vi "Nigel Tamagotchi Main.vi"() -> ()   [LabVIEW 2026]
uses:
  Type Defs/Queue Data.ctl
  Type Defs/Handler Data.ctl
panel:
  in  "Stop":bool
  out "Age (cycles)":u32
  out "Mood":string
  out "Cleanliness":i16(slide)=100 scale=0.0..100.0
  out "Energy":i16(slide)=100 scale=0.0..100.0
  out "Hunger":i16(slide) scale=0.0..100.0
  in  "Fixed Bug Button":bool
  in  "Broken Arrow Button":bool
  in  "Spagetti Button":bool
  in  "Sleep Button":bool
  in  "Clean Button":bool
  in  "Feed Button":bool
  out "Pict Ring":u16(ring)
  # "Nigel-gotchi (QMH)"
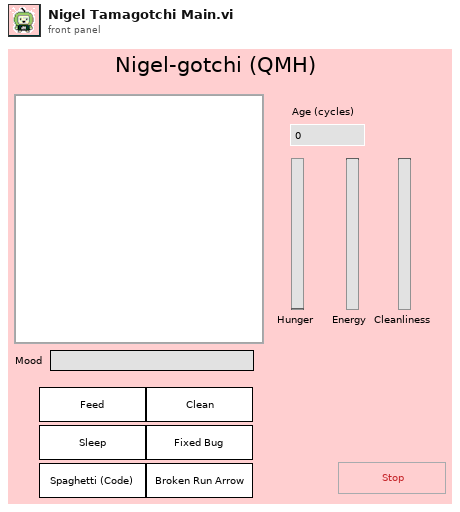
[diagram p1: front panel]
types:
  T1 = typedef "Queue Data.ctl" = cluster{"State":string, "Data":variant}
  T2 = typedef "Handler Data.ctl" = cluster{"Age (cycles)":u32, "Mood Override Counter":u32, "Mood Override":string, "Energy":i16, "Hunger":i16, "Cleanliness":i16}
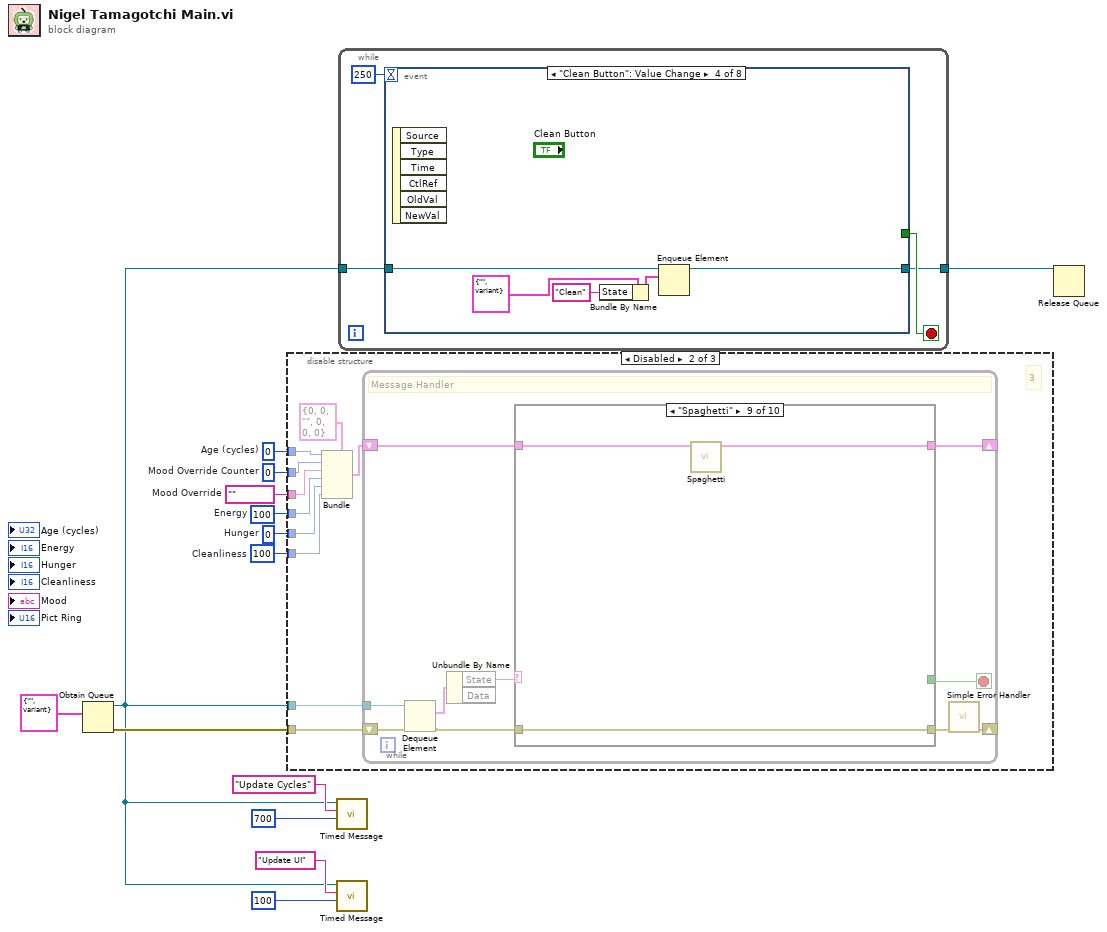
[diagram p0: block diagram]
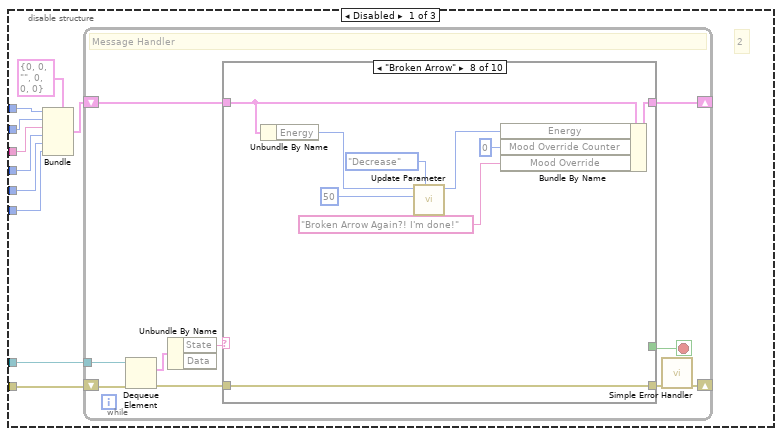
[diagram p2: hidden frame]
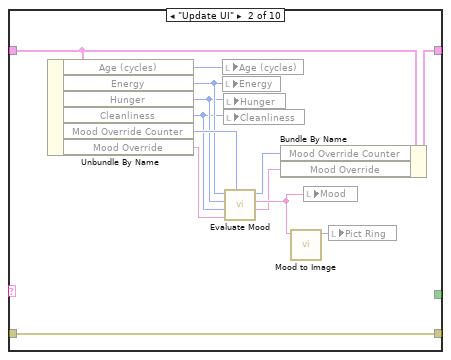
[diagram p4: hidden frame]
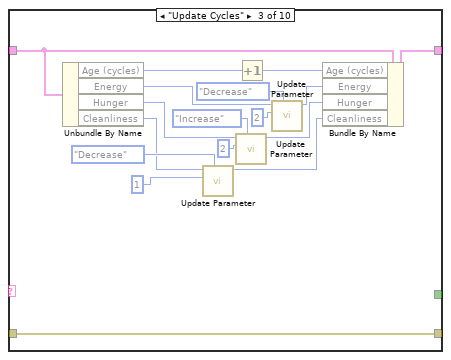
[diagram p5: hidden frame]
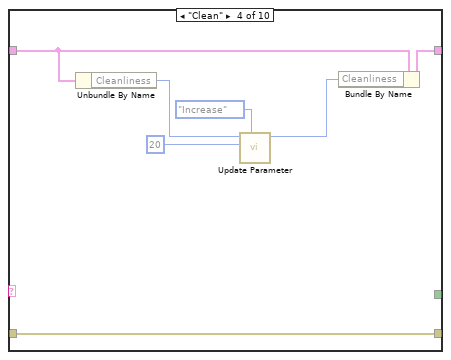
[diagram p6: hidden frame]
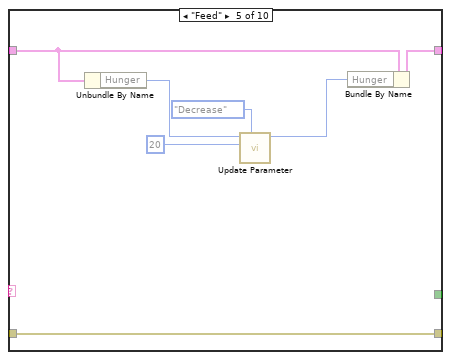
[diagram p7: hidden frame]
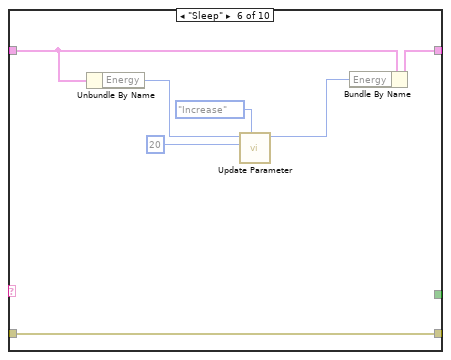
[diagram p8: hidden frame]
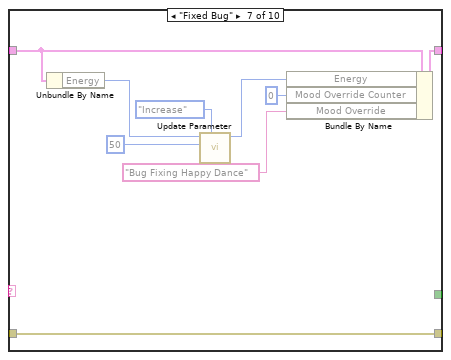
[diagram p9: hidden frame]
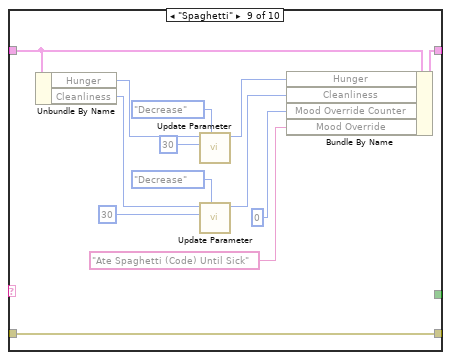
[diagram p10: hidden frame]
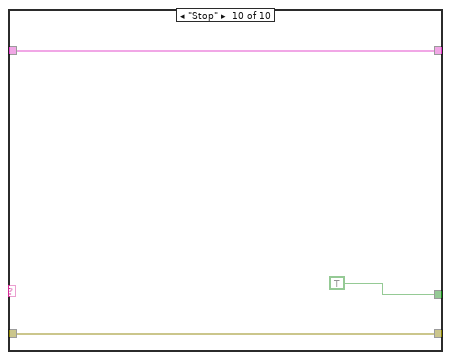
[diagram p11: hidden frame]
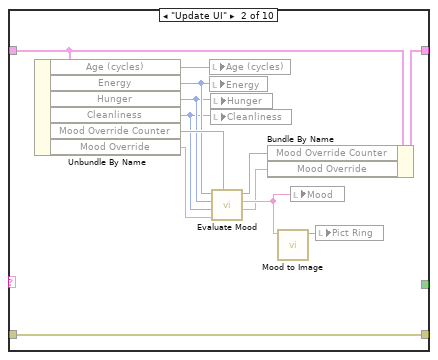
[diagram p13: hidden frame]
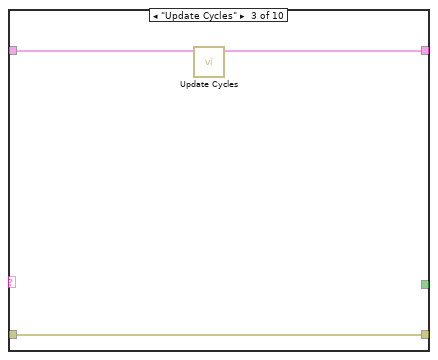
[diagram p14: hidden frame]
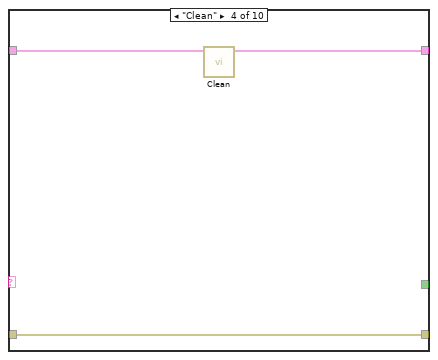
[diagram p15: hidden frame]
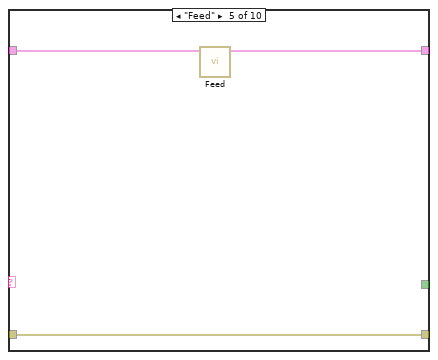
[diagram p16: hidden frame]
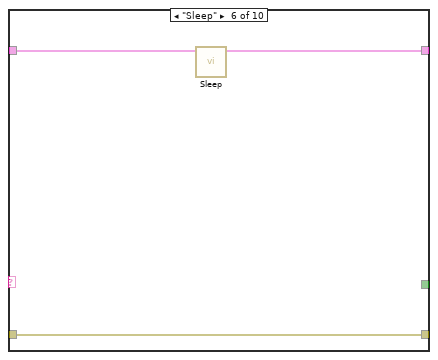
[diagram p17: hidden frame]
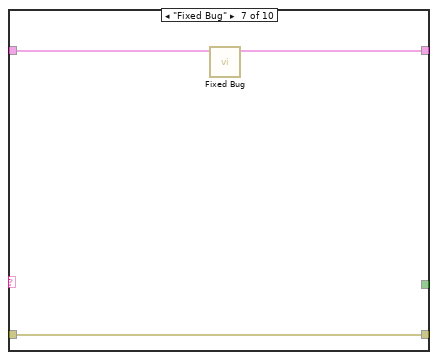
[diagram p18: hidden frame]
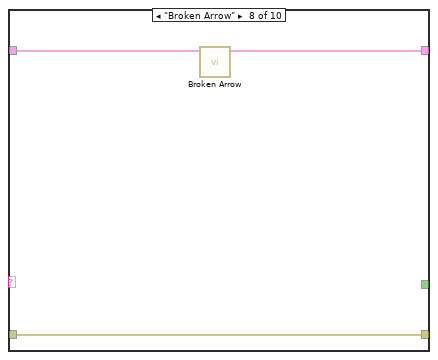
[diagram p19: hidden frame]
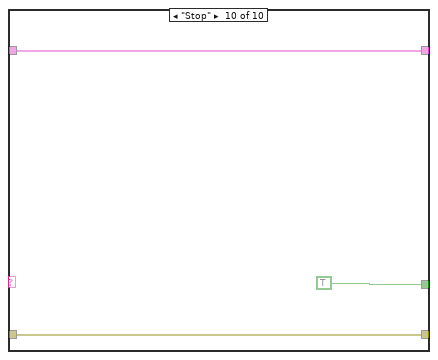
[diagram p20: hidden frame]
diagram:
  w7 = u32 0  # Mood Override Counter
  w10 = i16 100  # Energy
  w8 = i16 100  # Cleanliness
  w12 = u32 0  # Age (cycles)
  w9 = i16 0  # Hunger
  w11 = ""  # Mood Override
  n1 = Obtain Queue(element data type=T1 {"State"="", "Data"=variant}) -> (queue out=w1:refnum<queue>, error out=w13:errorcluster)  [unwired: 4 in, 1 out]
  n2 = disable-structure shown="Disabled" {
    disable-tunnel: w13 -> [w24 w131 w188]
    disable-tunnel: w12 -> [w22 w129 w187]
    disable-tunnel: w11 -> [w20 w127 w186]
    disable-tunnel: w10 -> [w19 w126 w185]
    disable-tunnel: w9 -> [w18 w125 w184]
    disable-tunnel: w8 -> [w17 w124 w183]
    disable-tunnel: w7 -> [w21 w128 w182]
    disable-tunnel: w1 -> [w23 w130 w181]
    frame Disabled {
      # "2"
      n3 = Bundle(cluster=T2 {"Age (cycles)"=0, "Mood Override Counter"=0, "Mood Override"="", "Energy"=0, "Hunger"=0, "Cleanliness"=0}, "Age (cycles)"=w22, "Mood Override Counter"=w21, "Mood Override"=w20, "Energy"=w19, "Hunger"=w18, "Cleanliness"=w17) -> (w16:T2)
      n4 = while {
        tunnel: w23 -> [w34]
        shift-right: [w29] -> _
        shift-left: w16 -> [w28]
        shift-right: [w25] -> _
        shift-left: w24 -> [w33]
        stop <- w30 stop-if-true
        # "Message Handler"
        n5 = Dequeue Element(queue=w34, error in (no error)=w33) -> (element=w32:T1, error out=w27:errorcluster)  [unwired: 1 in, 2 out]
        n6 = Unbundle By Name(w32) -> ("State"=w31:string)  [unwired: 1 out]
        n7 = case shown="\"Broken Arrow\"" w31 {
          tunnel: [_ _ _ _ _ _ _ _ _ TRUE] -> w30
          tunnel: [w36 w45 w58 w68 w75 w82 w91 w100 w113 w120] -> w29
          tunnel: w28 -> [w36 w47 w60 w70 w77 w84 w93 w102 w115 w120]
          tunnel: w27 -> [w35 w37 w50 w67 w74 w81 w88 w97 w106 w119]
          tunnel: [w35 w37 w50 w67 w74 w81 w88 w97 w106 w119] -> w26
          frame Default {
          }
          frame "Update UI" {
            # "Update UI (and cycles every tenth refresh)"
            n8 = Unbundle By Name(w47) -> ("Age (cycles)"=w46:u32, "Energy"=w40:i16, "Hunger"=w39:i16, "Cleanliness"=w38:i16, "Mood Override Counter"=w42:u32, "Mood Override"=w41:string)
            n9 = local write "Age (cycles)"(w46) -> ()
            n10 = local write "Energy"(w40) -> ()
            n11 = local write "Hunger"(w39) -> ()
            n12 = local write "Cleanliness"(w38) -> ()
            n13 = call "Evaluate Mood.vi"("Mood Override Counter"=w42, "Override Mood"=w41, "Cleanliness"=w38, "Hunger"=w39, "Energy"=w40) -> ("Mood Override"=w44:string, "Mood"=w49:string, "Mood Override Counter out"=w43:u32)  [unwired: 4 in]
            n14 = Bundle By Name(cluster=w47, "Mood Override Counter"=w43, "Mood Override"=w44) -> (w45:T2)
            n15 = call "Mood to Image.vi"("Mood"=w49) -> ("Image number"=w48:u16)  [unwired: 10 in]
            n16 = local write "Mood"(w49) -> ()
            n17 = local write "Pict Ring"(w48) -> ()
          }
          frame "Update Cycles" {
            n18 = Unbundle By Name(w60) -> ("Age (cycles)"=w59:u32, "Energy"=w56:i16, "Hunger"=w54:i16, "Cleanliness"=w52:i16)
            n19 = call "Update Parameter.vi"("Action"=enum16{"Increase", "Decrease"}."Decrease", "Modifier"=i16 1, "Parameter"=w52) -> ("New Value"=w51:i16)  [unwired: 8 in]
            n20 = call "Update Parameter.vi"("Action"=enum16{"Increase", "Decrease"}."Increase", "Modifier"=i16 2, "Parameter"=w54) -> ("New Value"=w53:i16)  [unwired: 8 in]
            n21 = Increment(x=w59) -> (x+1=w57:u32)
            n22 = call "Update Parameter.vi"("Action"=enum16{"Increase", "Decrease"}."Decrease", "Modifier"=i16 2, "Parameter"=w56) -> ("New Value"=w55:i16)  [unwired: 8 in]
            n23 = Bundle By Name(cluster=w60, "Age (cycles)"=w57, "Energy"=w55, "Hunger"=w53, "Cleanliness"=w51) -> (w58:T2)
          }
          frame "Clean" {
            # "Add 20, but make sure it doesn't go above 100 percent or below 0"
            n24 = Unbundle By Name(w70) -> ("Cleanliness"=w71:i16)
            n25 = call "Update Parameter.vi"("Action"=enum16{"Increase", "Decrease"}."Increase", "Modifier"=i16 20 ("y"), "Parameter"=w71) -> ("New Value"=w69:i16)  [unwired: 8 in]
            n26 = Bundle By Name(cluster=w70, "Cleanliness"=w69) -> (w68:T2)
          }
          frame "Feed" {
            # "Add 20, but make sure it doesn't go above 100 percent or below 0"
            n27 = Unbundle By Name(w77) -> ("Hunger"=w78:i16)
            n28 = call "Update Parameter.vi"("Action"=enum16{"Increase", "Decrease"}."Decrease", "Modifier"=i16 20 ("y"), "Parameter"=w78) -> ("New Value"=w76:i16)  [unwired: 8 in]
            n29 = Bundle By Name(cluster=w77, "Hunger"=w76) -> (w75:T2)
          }
          frame "Sleep" {
            # "Add 20, but make sure it doesn't go above 100 percent or below 0"
            n30 = Unbundle By Name(w84) -> ("Energy"=w85:i16)
            n31 = call "Update Parameter.vi"("Action"=enum16{"Increase", "Decrease"}."Increase", "Modifier"=i16 20 ("y"), "Parameter"=w85) -> ("New Value"=w83:i16)  [unwired: 8 in]
            n32 = Bundle By Name(cluster=w84, "Energy"=w83) -> (w82:T2)
          }
          frame "Fixed Bug" {
            n33 = Unbundle By Name(w93) -> ("Energy"=w94:i16)
            n34 = call "Update Parameter.vi"("Action"=enum16{"Increase", "Decrease"}."Increase", "Modifier"=i16 50 ("y"), "Parameter"=w94) -> ("New Value"=w92:i16)  [unwired: 8 in]
            n35 = Bundle By Name(cluster=w93, "Energy"=w92, "Mood Override Counter"=u32 0, "Mood Override"="Bug Fixing Happy Dance") -> (w91:T2)
          }
          frame "Broken Arrow" {
            n36 = Unbundle By Name(w102) -> ("Energy"=w103:i16)
            n37 = call "Update Parameter.vi"("Action"=enum16{"Increase", "Decrease"}."Decrease", "Modifier"=i16 50 ("y"), "Parameter"=w103) -> ("New Value"=w101:i16)  [unwired: 8 in]
            n38 = Bundle By Name(cluster=w102, "Energy"=w101, "Mood Override Counter"=u32 0, "Mood Override"="Broken Arrow Again?! I'm done!") -> (w100:T2)
          }
          frame "Spaghetti" {
            n39 = Unbundle By Name(w115) -> ("Hunger"=w116:i16, "Cleanliness"=w108:i16)
            n40 = call "Update Parameter.vi"("Action"=enum16{"Increase", "Decrease"}."Decrease", "Modifier"=i16 30 ("y"), "Parameter"=w116) -> ("New Value"=w114:i16)  [unwired: 8 in]
            n41 = call "Update Parameter.vi"("Action"=enum16{"Increase", "Decrease"}."Decrease", "Modifier"=i16 30 ("y"), "Parameter"=w108) -> ("New Value"=w107:i16)  [unwired: 8 in]
            n42 = Bundle By Name(cluster=w115, "Hunger"=w114, "Cleanliness"=w107, "Mood Override Counter"=u32 0, "Mood Override"="Ate Spaghetti (Code) Until Sick") -> (w113:T2)
          }
          frame "Stop" {
          }
        }
        n43 = call <vilib>:"Simple Error Handler.vi"("error in (no error)"=w26) -> ("error out"=w25:errorcluster)  [unwired: 4 in, 4 out]
      }
    }
    frame Disabled {
      # "3"
      n44 = Bundle(cluster=T2 {"Age (cycles)"=0, "Mood Override Counter"=0, "Mood Override"="", "Energy"=0, "Hunger"=0, "Cleanliness"=0}, "Age (cycles)"=w129, "Mood Override Counter"=w128, "Mood Override"=w127, "Energy"=w126, "Hunger"=w125, "Cleanliness"=w124) -> (w123:T2)
      n45 = while {
        tunnel: w130 -> [w141]
        shift-right: [w136] -> _
        shift-left: w123 -> [w135]
        shift-right: [w132] -> _
        shift-left: w131 -> [w140]
        stop <- w137 stop-if-true
        # "Message Handler"
        n46 = Dequeue Element(queue=w141, error in (no error)=w140) -> (element=w139:T1, error out=w133:errorcluster)  [unwired: 1 in, 2 out]
        n47 = Unbundle By Name(w139) -> ("State"=w138:string)  [unwired: 1 out]
        n48 = case shown="\"Spaghetti\"" w138 {
          tunnel: [_ _ _ _ _ _ _ _ _ TRUE] -> w137
          tunnel: [w143 w152 w158 w161 w164 w167 w170 w173 w175 w179] -> w136
          tunnel: w135 -> [w143 w154 w159 w162 w165 w168 w171 w174 w176 w179]
          tunnel: [w142 w144 w157 w160 w163 w166 w169 w172 w177 w178] -> w134
          tunnel: w133 -> [w142 w144 w157 w160 w163 w166 w169 w172 w177 w178]
          frame Default {
          }
          frame "Update UI" {
            # "Update UI (and cycles every tenth refresh)"
            n49 = Unbundle By Name(w154) -> ("Age (cycles)"=w153:u32, "Energy"=w147:i16, "Hunger"=w146:i16, "Cleanliness"=w145:i16, "Mood Override Counter"=w149:u32, "Mood Override"=w148:string)
            n50 = local write "Age (cycles)"(w153) -> ()
            n51 = local write "Energy"(w147) -> ()
            n52 = local write "Hunger"(w146) -> ()
            n53 = local write "Cleanliness"(w145) -> ()
            n54 = call "Evaluate Mood.vi"("Mood Override Counter"=w149, "Override Mood"=w148, "Cleanliness"=w145, "Hunger"=w146, "Energy"=w147) -> ("Mood Override"=w151:string, "Mood"=w156:string, "Mood Override Counter out"=w150:u32)  [unwired: 4 in]
            n55 = Bundle By Name(cluster=w154, "Mood Override Counter"=w150, "Mood Override"=w151) -> (w152:T2)
            n56 = call "Mood to Image.vi"("Mood"=w156) -> ("Image number"=w155:u16)  [unwired: 10 in]
            n57 = local write "Mood"(w156) -> ()
            n58 = local write "Pict Ring"(w155) -> ()
          }
          frame "Update Cycles" {
            n59 = call "Update Cycles.vi"("cluster in"=w159) -> ("cluster out"=w158:T2)  [unwired: 10 in]
          }
          frame "Clean" {
            # "Add 20, but make sure it doesn't go above 100 percent or below 0"
            n60 = call "Clean.vi"("cluster in"=w162) -> ("cluster out"=w161:T2)  [unwired: 10 in]
          }
          frame "Feed" {
            # "Add 20, but make sure it doesn't go above 100 percent or below 0"
            n61 = call "Feed.vi"("cluster in"=w165) -> ("cluster out"=w164:T2)  [unwired: 10 in]
          }
          frame "Sleep" {
            # "Add 20, but make sure it doesn't go above 100 percent or below 0"
            n62 = call "Sleep.vi"("cluster in"=w168) -> ("cluster out"=w167:T2)  [unwired: 10 in]
          }
          frame "Fixed Bug" {
            n63 = call "Fixed Bug.vi"("cluster in"=w171) -> ("cluster out"=w170:T2)  [unwired: 10 in]
          }
          frame "Broken Arrow" {
            n64 = call "Broken Arrow.vi"("cluster in"=w174) -> ("cluster out"=w173:T2)  [unwired: 10 in]
          }
          frame "Spaghetti" {
            n65 = call "Spaghetti.vi"("cluster in"=w176) -> ("cluster out"=w175:T2)  [unwired: 10 in]
          }
          frame "Stop" {
          }
        }
        n66 = call <vilib>:"Simple Error Handler.vi"("error in (no error)"=w134) -> ("error out"=w132:errorcluster)  [unwired: 4 in, 4 out]
      }
    }
    frame Enabled {
      # "1"
      n67 = while {
        tunnel: w181 -> [w208]
        shift-right: [w203] -> _
        shift-left: w187 -> [w202]
        shift-right: [w201] -> _
        shift-left: w186 -> [w200]
        shift-right: [w199] -> _
        shift-left: w185 -> [w198]
        shift-right: [w197] -> _
        shift-left: w184 -> [w196]
        shift-right: [w195] -> _
        shift-left: w183 -> [w194]
        shift-right: [w193] -> _
        shift-left: w182 -> [w192]
        shift-right: [w189] -> _
        shift-left: w188 -> [w207]
        stop <- w204 stop-if-true
        # "Message Handler"
        n68 = Dequeue Element(queue=w208, error in (no error)=w207) -> (element=w206:T1, error out=w191:errorcluster)  [unwired: 1 in, 2 out]
        n69 = Unbundle By Name(w206) -> ("State"=w205:string)  [unwired: 1 out]
        n70 = case shown="\"Broken Arrow\"" w205 {
          tunnel: [_ _ _ _ _ _ _ _ _ TRUE] -> w204
          tunnel: [w215 w222 w248 w265 w275 w285 w295 w305 w318 w325] -> w203
          tunnel: w202 -> [w215 w222 w249 w265 w275 w285 w295 w305 w318 w325]
          tunnel: [w214 w223 w247 w264 w274 w284 "Bug Fixing Happy Dance" ("Mood Override") "Broken Arrow Again?! I'm done!" ("Mood Override") "Ate Spaghetti (Code) Until Sick" ("Mood Override") w324] -> w201
          tunnel: w200 -> [w214 w226 w247 w264 w274 w284 _ _ _ w324]
          tunnel: [w213 w218 w239 w263 w271 w280 w290 w300 w314 w323] -> w199
          tunnel: w198 -> [w213 w218 w238 w263 w271 w281 w292 w302 w314 w323]
          tunnel: [w212 w217 w235 w262 w272 w282 w294 w304 w312 w322] -> w197
          tunnel: w196 -> [w212 w217 w236 w262 w270 w282 w294 w304 w313 w322]
          tunnel: [w211 w221 w232 w260 w273 w283 w293 w303 w310 w321] -> w195
          tunnel: w194 -> [w211 w221 w231 w261 w273 w283 w293 w303 w311 w321]
          tunnel: [w210 w224 w246 w258 w268 w278 u32 0 ("Mood Override Counter") u32 0 ("Mood Override Counter") u32 0 ("Mood Override Counter") w320] -> w193
          tunnel: w192 -> [w210 w225 w246 w258 w268 w278 _ _ _ w320]
          tunnel: w191 -> [w209 w216 w227 w256 w266 w276 w286 w296 w306 w319]
          tunnel: [w209 w216 w227 w256 w266 w276 w286 w296 w306 w319] -> w190
          frame Default {
          }
          frame "Update UI" {
            # "Update UI (and cycles every tenth refresh)"
            n71 = local write "Age (cycles)"(w222) -> ()
            n72 = local write "Energy"(w218) -> ()
            n73 = local write "Hunger"(w217) -> ()
            n74 = local write "Cleanliness"(w221) -> ()
            n75 = call "Evaluate Mood.vi"("Mood Override Counter"=w225, "Override Mood"=w226, "Cleanliness"=w221, "Hunger"=w217, "Energy"=w218) -> ("Mood Override"=w223:string, "Mood"=w220:string, "Mood Override Counter out"=w224:u32)  [unwired: 4 in]
            n76 = call "Mood to Image.vi"("Mood"=w220) -> ("Image number"=w219:u16)  [unwired: 10 in]
            n77 = local write "Mood"(w220) -> ()
            n78 = local write "Pict Ring"(w219) -> ()
          }
          frame "Update Cycles" {
            n79 = property on="Pict Ring" class="Ring (strict)"() -> ("Top"=w242:i32)  [unwired: 2 in, 2 out]
            n80 = Increment(x=w249) -> (x+1=w248:u32)
            n81 = call "Update Parameter.vi"("Action"=enum16{"Increase", "Decrease"}."Decrease", "Modifier"=i16 1, "Parameter"=w231) -> ("New Value"=w232:i16)  [unwired: 8 in]
            n82 = Quotient & Remainder(x=w242, y=2) -> (x-y*floor(x/y)=w244:i32)  [unwired: 1 out]
            n83 = Equal To 0?(x=w244) -> (x = 0?=w243:bool)
            n84 = call "Update Parameter.vi"("Action"=enum16{"Increase", "Decrease"}."Increase", "Modifier"=i16 2, "Parameter"=w236) -> ("New Value"=w235:i16)  [unwired: 8 in]
            n85 = case shown="False" w243 {
              tunnel: w242 -> [w252 w255]
              tunnel: 3 ("y") -> [w251 w254]
              tunnel: [w250 w253] -> w240
              frame False {
                n86 = Add(x=w252, y=w251) -> (x+y=w250:i32)
              }
              frame True {
                n87 = Subtract(x=w255, y=w254) -> (x-y=w253:i32)
              }
            }
            n88 = call "Update Parameter.vi"("Action"=enum16{"Increase", "Decrease"}."Decrease", "Modifier"=i16 2, "Parameter"=w238) -> ("New Value"=w239:i16)  [unwired: 8 in]
            n89 = property on="Pict Ring" class="Ring (strict)"("Top"=w240) -> ()  [unwired: 2 in, 2 out]
          }
          frame "Clean" {
            # "Add 20, but make sure it doesn't go above 100 percent or below 0"
            n90 = call "Update Parameter.vi"("Action"=enum16{"Increase", "Decrease"}."Increase", "Modifier"=i16 20 ("y"), "Parameter"=w261) -> ("New Value"=w260:i16)  [unwired: 8 in]
          }
          frame "Feed" {
            # "Subtract 20 from hunger, but make sure it doesn't go above 100 or below 0"
            n91 = call "Update Parameter.vi"("Action"=enum16{"Increase", "Decrease"}."Decrease", "Modifier"=i16 20 ("y"), "Parameter"=w270) -> ("New Value"=w272:i16)  [unwired: 8 in]
          }
          frame "Sleep" {
            n92 = call "Update Parameter.vi"("Action"=enum16{"Increase", "Decrease"}."Increase", "Modifier"=i16 20 ("y"), "Parameter"=w281) -> ("New Value"=w280:i16)  [unwired: 8 in]
          }
          frame "Fixed Bug" {
            n93 = call "Update Parameter.vi"("Action"=enum16{"Increase", "Decrease"}."Increase", "Modifier"=i16 50, "Parameter"=w292) -> ("New Value"=w290:i16)  [unwired: 8 in]
          }
          frame "Broken Arrow" {
            n94 = call "Update Parameter.vi"("Action"=enum16{"Increase", "Decrease"}."Decrease", "Modifier"=i16 50, "Parameter"=w302) -> ("New Value"=w300:i16)  [unwired: 8 in]
          }
          frame "Spaghetti" {
            n95 = call "Update Parameter.vi"("Action"=enum16{"Increase", "Decrease"}."Decrease", "Modifier"=i16 30, "Parameter"=w313) -> ("New Value"=w312:i16)  [unwired: 8 in]
            n96 = call "Update Parameter.vi"("Action"=enum16{"Increase", "Decrease"}."Decrease", "Modifier"=i16 30, "Parameter"=w311) -> ("New Value"=w310:i16)  [unwired: 8 in]
          }
          frame "Stop" {
          }
        }
        n97 = call <vilib>:"Simple Error Handler.vi"("error in (no error)"=w190) -> ("error out"=w189:errorcluster)  [unwired: 4 in, 4 out]
      }
    }
  }
  n98 = call "Timed Message.vi"("Interval (ms)"=u32 700 ("milliseconds to wait"), "State"="Update Cycles", "Queue in"=w1) -> ()  [unwired: 9 in]
  n99 = call "Timed Message.vi"("Interval (ms)"=u32 100 ("milliseconds to wait"), "State"="Update UI", "Queue in"=w1) -> ()  [unwired: 9 in]
  n100 = while {
    tunnel: w1 -> [w329]
    tunnel: [w328] -> w6
    stop <- w330 stop-if-true
    n101 = event shown="[3] \"Clean Button\": Value Change" {
      selector: _ -> [_ _ _ _ _ _ _ _]
      dyn-events: _ -> [_ _ _ _ _ _ _ _]
      timeout: 250 -> [_ _ _ _ _ _ _ _]
      tunnel: [_ "Stop" _ _ _ _ _ _] -> w330
      tunnel: w329 -> [w337 w348 w351 w356 w361 w366 w371 w376]
      tunnel: [w337 w344 w350 w355 w360 w365 w370 w375] -> w328
      event Timeout {
        n102 = event-data() -> ()  [unwired: 1 in, 1 out]
        n103 = property on="Pict Ring" class="Ring (strict)"() -> ("Top"=w335:i32)  [unwired: 2 in, 2 out]
        n104 = Quotient & Remainder(x=w335, y=2) -> (x-y*floor(x/y)=w333:i32)  [unwired: 1 out]
        n105 = Equal To 0?(x=w333) -> (x = 0?=w334:bool)
        n106 = case shown="False" w334 {
          tunnel: w335 -> [w340 w343]
          tunnel: 3 ("y") -> [w339 w342]
          tunnel: [w338 w341] -> w336
          frame False {
            n107 = Add(x=w340, y=w339) -> (x+y=w338:i32)
          }
          frame True {
            n108 = Subtract(x=w343, y=w342) -> (x-y=w341:i32)
          }
        }
        n109 = property on="Pict Ring" class="Ring (strict)"("Top"=w336) -> ()  [unwired: 2 in, 2 out]
      }
      event "Stop": Value Change {
        n110 = event-data() -> ()  [unwired: 1 in, 6 out]
        n111 = Bundle By Name(cluster=T1 {"State"="", "Data"=variant} ("element"), "State"="Stop") -> (w346:T1)
        n112 = Enqueue Element(queue=w348, element=w346) -> (queue out=w344:refnum<queue>)  [unwired: 2 in, 2 out]
      }
      event "Feed Button": Value Change {
        n113 = event-data() -> ()  [unwired: 1 in, 6 out]
        n114 = Bundle By Name(cluster=T1 {"State"="", "Data"=variant} ("element"), "State"="Feed") -> (w353:T1)
        n115 = Enqueue Element(queue=w351, element=w353) -> (queue out=w350:refnum<queue>)  [unwired: 2 in, 2 out]
      }
      event "Clean Button": Value Change {
        n116 = event-data() -> ()  [unwired: 1 in, 6 out]
        n117 = Bundle By Name(cluster=T1 {"State"="", "Data"=variant} ("element"), "State"="Clean") -> (w358:T1)
        n118 = Enqueue Element(queue=w356, element=w358) -> (queue out=w355:refnum<queue>)  [unwired: 2 in, 2 out]
      }
      event "Sleep Button": Value Change {
        n119 = event-data() -> ()  [unwired: 1 in, 6 out]
        n120 = Bundle By Name(cluster=T1 {"State"="", "Data"=variant} ("element"), "State"="Sleep") -> (w363:T1)
        n121 = Enqueue Element(queue=w361, element=w363) -> (queue out=w360:refnum<queue>)  [unwired: 2 in, 2 out]
      }
      event "Spagetti Button": Value Change {
        n122 = event-data() -> ()  [unwired: 1 in, 6 out]
        n123 = Bundle By Name(cluster=T1 {"State"="", "Data"=variant} ("element"), "State"="Spaghetti") -> (w369:T1)
        n124 = Enqueue Element(queue=w366, element=w369) -> (queue out=w365:refnum<queue>)  [unwired: 2 in, 2 out]
      }
      event "Broken Arrow Button": Value Change {
        n125 = event-data() -> ()  [unwired: 1 in, 6 out]
        n126 = Bundle By Name(cluster=T1 {"State"="", "Data"=variant} ("element"), "State"="Broken Arrow") -> (w373:T1)
        n127 = Enqueue Element(queue=w371, element=w373) -> (queue out=w370:refnum<queue>)  [unwired: 2 in, 2 out]
      }
      event "Fixed Bug Button": Value Change {
        n128 = event-data() -> ()  [unwired: 1 in, 6 out]
        n129 = Bundle By Name(cluster=T1 {"State"="", "Data"=variant} ("element"), "State"="Fixed Bug") -> (w378:T1)
        n130 = Enqueue Element(queue=w376, element=w378) -> (queue out=w375:refnum<queue>)  [unwired: 2 in, 2 out]
      }
    }
  }
  n131 = Release Queue(queue=w6) -> ()  [unwired: 2 in, 3 out]
